vi "ReadLastTimestamp.vi"(8 "error in (no error)":errorcluster, 10 "Terminal":string, 11 "instrument handle":refnum<k15>) -> (0 "error out":errorcluster, 2 "time stamp out":timestamp, 3 "instrument handle out":refnum<k15>)   [LabVIEW 2018, in "DigitizerPlugins.lvlib" / "NiDaqMx.lvclass"]
uses:
  NiDaqMx.lvclass
  <instrlib>/niSync/niSync.llb/niSync Read Trigger Time Stamp (Single).vi
panel:
  out "Edges":enum32{"rising", "falling"}[](array[ring])
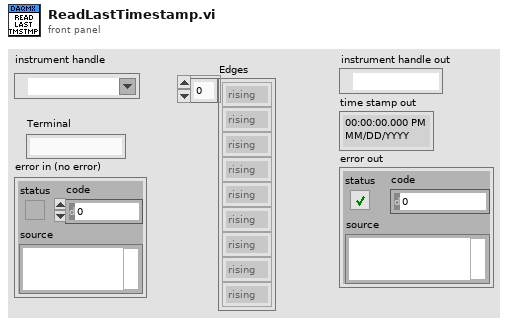
[diagram p1: front panel]
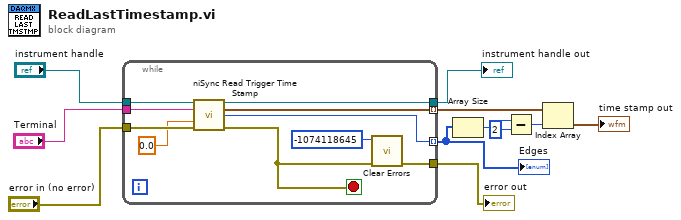
[diagram p0: block diagram]
diagram:
  n1 = while {
    tunnel: "instrument handle" -> [w21]
    tunnel: "Terminal" -> [w20]
    tunnel: "error in (no error)" -> [w19]
    tunnel: [w17] -> w6 mode=indexing
    tunnel: [w16] -> w8
    tunnel: [w15] -> w4 mode=indexing
    tunnel: [w12] -> w7
    stop <- w14 stop-if-true
    n2 = call-poly <instrlib>:"niSync Read Trigger Time Stamp.vi"("instrument handle"=w21, "terminal"=w20, "timeout"=0.0, "error in (no error)"=w19) -> ("instrument handle out"=w16:refnum<k15>, "time stamp out"=w17:timestamp, "detected edge"=w15:enum32{"rising", "falling"}, "error out"=w14:errorcluster)  [unwired: 8 in]
    n3 = call <vilib>:"Clear Errors.vi"("error in (no error)"=w14, "specific error code to clear (0: all)"=-1074118645) -> ("error out"=w12:errorcluster)  [unwired: 4 in, 1 out]
  }
  "instrument handle out" <- w8
  "error out" <- w7
  "Edges" <- w4
  n4 = Array Size(array=w4) -> (size(s)=w2:i32)
  n5 = Subtract(x=w2, y=2) -> (x-y=w3:i32)
  n6 = Index Array(array=w6, index=w3) -> (element=→"time stamp out":timestamp)
